vi "acquisitionStartStop.vi"(1 "acquisitionDuration (ms)":u32) -> ()   [LabVIEW 2017]
doc: "Sets acquisitionStart to true, waits for acquisitionDuration, and sets acquisitionStop to true (and acquisitionStart to false)."
uses:
  globalUtilities.vi
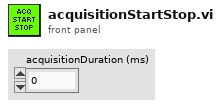
[diagram p1: front panel]
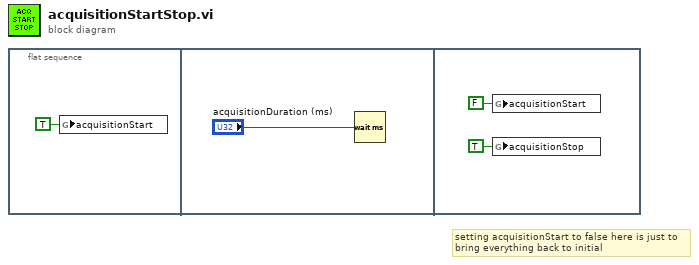
[diagram p0: block diagram]
diagram:
  # "setting acquisitionStart to false here is just to\nbring everything back to initial"
  n1 = flat-sequence {
    frame #0 {
      n2 = global write "globalUtilities.vi" "acquisitionStart"(TRUE ("acquisitionStart")) -> ()
    }
    frame #1 {
      n3 = Wait (ms)(milliseconds to wait="acquisitionDuration (ms)") -> ()  [unwired: 1 out]
    }
    frame #2 {
      n4 = global write "globalUtilities.vi" "acquisitionStart"(FALSE ("acquisitionStart")) -> ()
      n5 = global write "globalUtilities.vi" "acquisitionStop"(TRUE ("acquisitionStart")) -> ()
    }
  }
